vi "Get All Methods from LVObject.vi"(8 "error in":errorcluster, 10 "LabVIEW Object":refnum<class>) -> (0 "error out":errorcluster, 2 "Methods":path[](array[path]))   [LabVIEW 2013, in "VITesterUtilities.lvlib"]
uses:
  Libraries/VITesterUtilities.lvlib
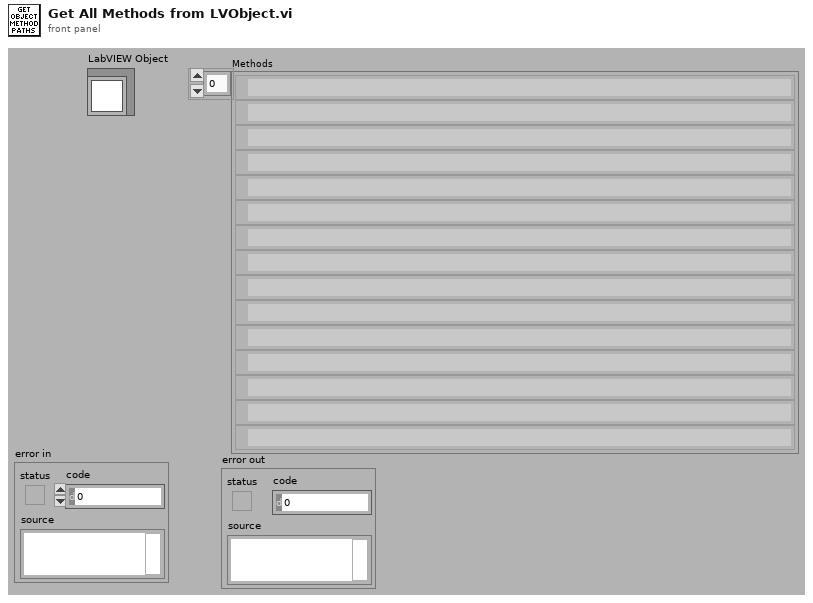
[diagram p1: front panel]
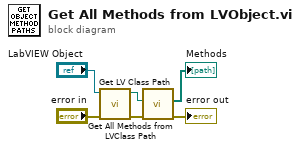
[diagram p0: block diagram]
diagram:
  n1 = call <vilib>:"Get LV Class Path.vi"("error in (no error)"="error in", "object"="LabVIEW Object") -> ("error out"=w3:errorcluster, "class path"=w5:path)  [unwired: 8 in]
  n2 = call "Get All Methods from LVClass Path.vi"("error in"=w3, "class path"=w5) -> ("error out"=→"error out":errorcluster, "Methods"=→"Methods":path[])  [unwired: 8 in]
